vi "SIM ChkFixedTimesteps.vi"(4 "Clock Rate (Hz)":u32, 6 "Calculate using Time Step":bool, 7 "MachineEpsilon":dbl, 8 "Error In":errorcluster, 9 "Automatic Discrete Step Size?":bool, 10 "DiscreteTimeStep":dbl, 11 "TimeStep":dbl) -> (0 "Error Out":errorcluster)   [LabVIEW 2014]
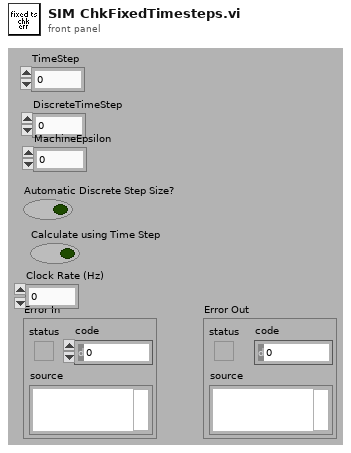
[diagram p1: front panel]
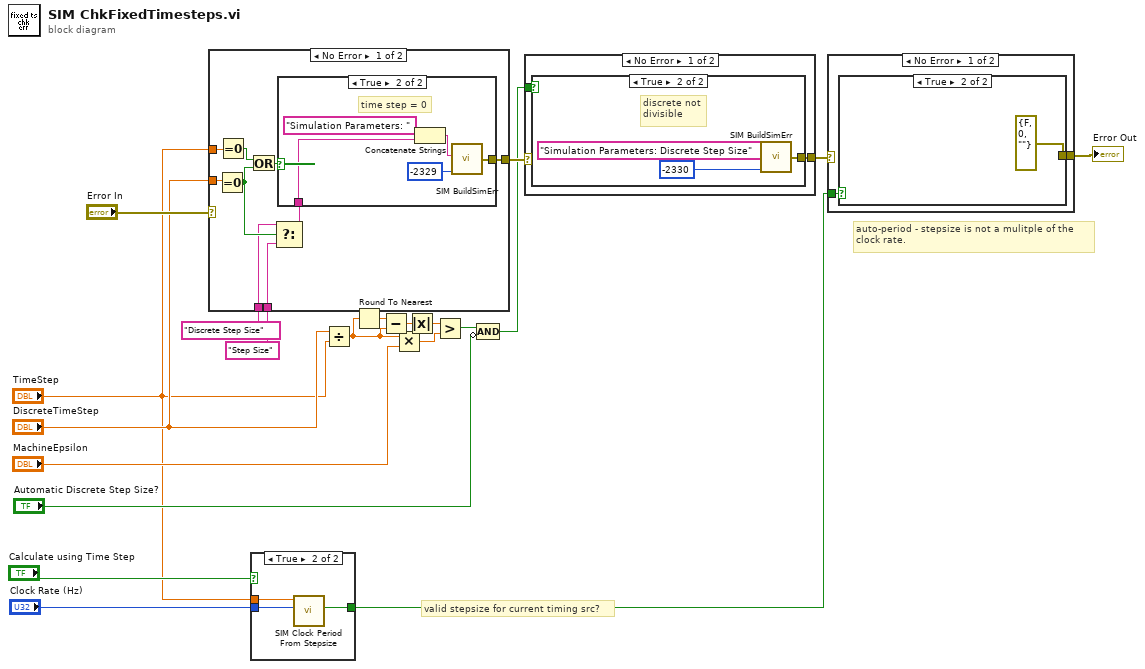
[diagram p0: block diagram]
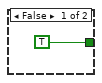
[diagram p2: hidden frame]
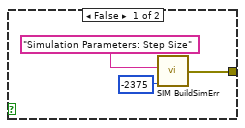
[diagram p3: hidden frame]
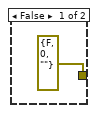
[diagram p5: hidden frame]
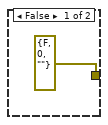
[diagram p7: hidden frame]
diagram:
  # "valid stepsize for current timing src?"
  # "auto-period - stepsize is not a mulitple of the\nclock rate."
  n1 = case shown="No Error" "Error In" {
    selector: "Error In" -> [_ w36]
    tunnel: [w29 w36] -> w17
    tunnel: "DiscreteTimeStep" -> [w28 _]
    tunnel: "TimeStep" -> [w27 _]
    tunnel: "Discrete Step Size" ("Additional Details") -> [w23 _]
    tunnel: "Step Size" ("Additional Details") -> [w22 _]
    frame No Error {
      n2 = Equal To 0?(x=w28) -> (x = 0?=w24:bool)
      n3 = Equal To 0?(x=w27) -> (x = 0?=w26:bool)
      n4 = Or(x=w26, y=w24) -> (x .or. y?=w25:bool)
      n5 = Select(t=w23, s=w24, f=w22) -> (s? t:f=w21:string)
      n6 = case shown="True" w25 {
        tunnel: [errorcluster {"status"=FALSE, "code"=0, "source"=""} ("Error Cluster") w35] -> w29
        tunnel: w21 -> [_ w32]
        frame False {
        }
        frame True {
          # "time step = 0"
          n7 = Concatenate Strings("Simulation Parameters: " ("CallChain"), w32) -> (w31:string)
          n8 = call "SIM BuildSimErr.vi"("error.code"=-2329, "Block Name"=w31) -> ("Error Cluster"=w35:errorcluster)  [unwired: 2 in]
        }
      }
    }
    frame Error {
    }
  }
  n9 = case shown="True" "Calculate using Time Step" {
    tunnel: "Clock Rate (Hz)" -> [_ w38]
    tunnel: "TimeStep" -> [_ w40]
    tunnel: [TRUE ("Valid?") w39] -> w2
    frame False {
    }
    frame True {
      n10 = call "SIM Clock Period From Stepsize.vi"("Clock Rate (Hz)"=w38, "Step Size"=w40) -> ("Valid?"=w39:bool)  [unwired: 8 in, 1 out]
    }
  }
  n11 = Divide(x="DiscreteTimeStep", y="TimeStep") -> (x/y=w13:dbl)
  n12 = Round To Nearest(number=w13) -> (nearest integer value=w16:dbl)
  n13 = Subtract(x=w16, y=w13) -> (x-y=w14:dbl)
  n14 = Multiply(x=w13, y="MachineEpsilon") -> (x*y=w12:dbl)
  n15 = Absolute Value(x=w14) -> (abs(x)=w15:dbl)
  n16 = Greater?(x=w15, y=w12) -> (0:w9:bool)
  n17 = Compound Arithmetic op=AND(w9, invert "Automatic Discrete Step Size?") -> (w7:bool)
  n18 = case shown="No Error" w17 {
    selector: w17 -> [_ w47]
    tunnel: [w41 w47] -> w6
    tunnel: w7 -> [w42 _]
    frame No Error {
      n19 = case shown="True" w42 {
        tunnel: [errorcluster {"status"=FALSE, "code"=0, "source"=""} ("Error Cluster") w45] -> w41
        frame False {
        }
        frame True {
          # "discrete not\ndivisible"
          n20 = call "SIM BuildSimErr.vi"("error.code"=-2330, "Block Name"="Simulation Parameters: Discrete Step Size" ("CallChain")) -> ("Error Cluster"=w45:errorcluster)  [unwired: 2 in]
        }
      }
    }
    frame Error {
    }
  }
  n21 = case shown="No Error" w6 {
    selector: w6 -> [_ w54]
    tunnel: [w49 w54] -> w1
    tunnel: w2 -> [w48 _]
    frame No Error {
      n22 = case shown="True" w48 {
        tunnel: [w51 errorcluster {"status"=FALSE, "code"=0, "source"=""} ("Error Cluster")] -> w49
        frame False {
          n23 = call "SIM BuildSimErr.vi"("error.code"=-2375, "Block Name"="Simulation Parameters: Step Size" ("CallChain")) -> ("Error Cluster"=w51:errorcluster)  [unwired: 2 in]
        }
        frame True {
        }
      }
    }
    frame Error {
    }
  }
  "Error Out" <- w1
